vi "Metronome.vi"(8 "error in (no error)":errorcluster, 9 "MetronomeData":T2={"Interval"=250, "Message"="Tick"}, 10 "Queue in (write)":T1, 11 "Queue in (read)":T1) -> (0 "error out":errorcluster, 2 "Queue out (write)":T1, 3 "Queue out (read)":T1)   [LabVIEW 2020]
doc: "This VI enqueues a message with specified time interval in Queue in (write) queue. \nIt requires two refnums to queues made with CreateMessageQueue.vi. \nIt reads messages from Queue in (read). Valid messages: Start, Set, Pause, Stop. \nStart - begin or resume operations; Set - new interval (integer) provided as data with a message; Pause - halt operations and wait; Stop - stop VI.\nCluster MetronomeData provides an initial interval and text of the message to be send out in Queue in (write)."
uses:
  MetronomeData.ctl
  MessageQueue/QueueRef.ctl
  <vilib>/Utility/error.llb/Error Cluster From Error Code.vi
  <vilib>/ErrorRing/Error Ring.xnode
  MessageQueue/MessageQueue.lvlib
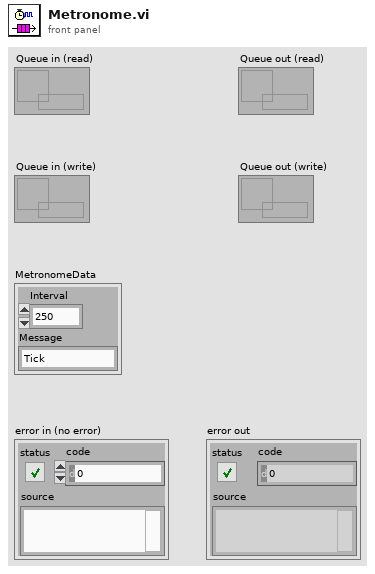
[diagram p1: front panel]
types:
  T1 = typedef "MessageQueue.lvlib/QueueRef.ctl" = refnum<queue>
  T2 = typedef "MetronomeData.ctl" = cluster{"Interval":i32, "Message":string}
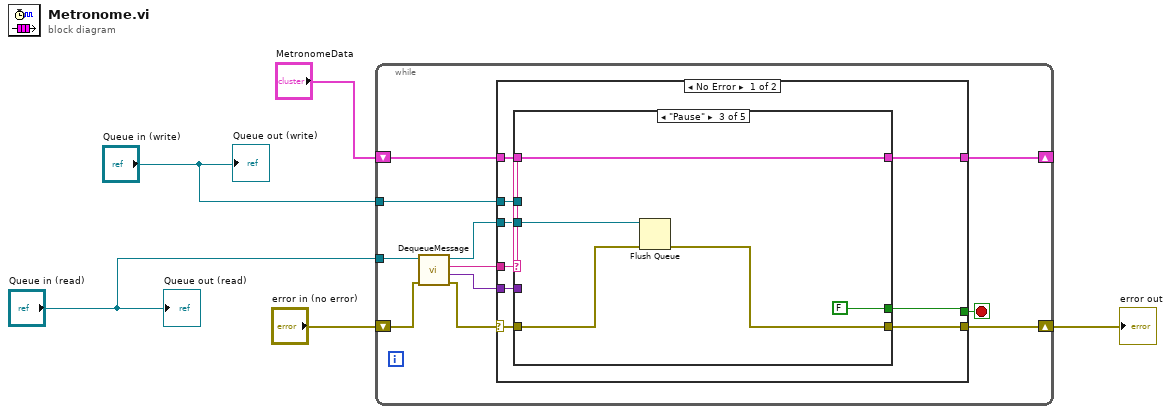
[diagram p0: block diagram]
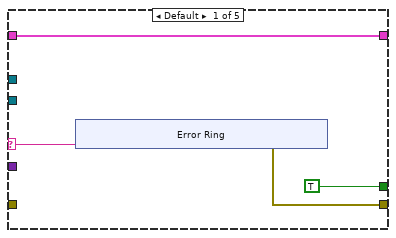
[diagram p2: hidden frame]
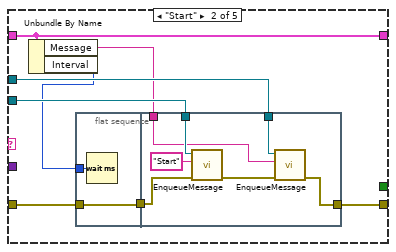
[diagram p3: hidden frame]
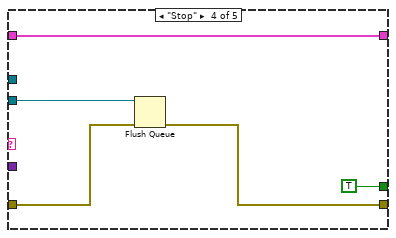
[diagram p4: hidden frame]
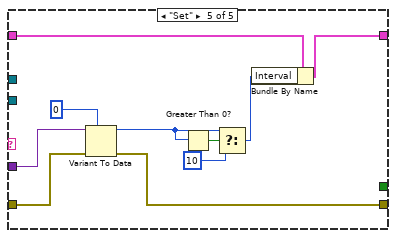
[diagram p5: hidden frame]
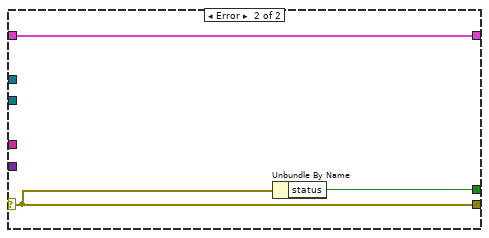
[diagram p6: hidden frame]
diagram:
  n1 = while {
    tunnel: "Queue in (read)" -> [w11]
    tunnel: "Queue in (write)" -> [w12]
    shift-right: [w15] -> _
    shift-left: "MetronomeData" -> [w16]
    shift-right: [w14] -> w4
    shift-left: "error in (no error)" -> [w7]
    stop <- w13 stop-if-true
    n2 = call "DequeueMessage.vi"("error in (no error)"=w7, "queue in"=w11) -> ("error out"=w6:errorcluster, "Data (Variant)"=w10:variant, "Message"=w9:string, "queue out (copy)"=w8:T1)  [unwired: 6 in]
    n3 = case shown="No Error" w6 {
      selector: w6 -> [w24 w75]
      tunnel: w16 -> [w23 w76]
      tunnel: [w22 w76] -> w15
      tunnel: [w25 w75] -> w14
      tunnel: [w20 w74] -> w13
      tunnel: w12 -> [w21 _]
      tunnel: w10 -> [w19 _]
      tunnel: w9 -> [w18 _]
      tunnel: w8 -> [w17 _]
      frame No Error {
        n4 = case shown="\"Pause\"" w18 {
          selector: w18 -> [w26 _ _ _ _]
          tunnel: [w27 w43 w56 w59 w67] -> w25
          tunnel: w24 -> [_ w37 w57 w62 w71]
          tunnel: w23 -> [w29 w41 w55 w61 w66]
          tunnel: [w29 w41 w55 w61 w65] -> w22
          tunnel: w17 -> [_ w44 w58 w63 _]
          tunnel: w21 -> [_ w42 _ _ _]
          tunnel: w19 -> [_ _ _ _ w73]
          tunnel: [TRUE _ FALSE TRUE _] -> w20
          frame Default {
            n5 = xnode "Error Ring"("parameter 0"=w26) -> ("error out"=w27:errorcluster)
          }
          frame "Start" {
            n6 = Unbundle By Name(w41) -> ("Message"=w39:string, "Interval"=w40:i32)
            n7 = flat-sequence {
              tunnel: w40 -> [w46]
              tunnel: [w45] -> w38
              tunnel: w37 -> [w45]
              tunnel: w44 -> [w52]
              tunnel: [w49] -> w43
              tunnel: w42 -> [w51]
              tunnel: w39 -> [w48]
              tunnel: w38 -> [w47]
              frame #0 {
                n8 = Wait (ms)(milliseconds to wait=w46) -> ()  [unwired: 1 out]
              }
              frame #1 {
                n9 = call "EnqueueMessage.vi"("error in (no error)"=w47, "Message"="Start", "queue in"=w52) -> ("error out"=w50:errorcluster)  [unwired: 7 in, 1 out]
                n10 = call "EnqueueMessage.vi"("error in (no error)"=w50, "Message"=w48, "queue in"=w51) -> ("error out"=w49:errorcluster)  [unwired: 7 in, 1 out]
              }
            }
          }
          frame "Pause" {
            n11 = Flush Queue(queue=w58, error in (no error)=w57) -> (error out=w56:errorcluster)  [unwired: 2 out]
          }
          frame "Stop" {
            n12 = Flush Queue(queue=w63, error in (no error)=w62) -> (error out=w59:errorcluster)  [unwired: 2 out]
          }
          frame "Set" {
            n13 = Variant To Data(error in=w71, type=0, Variant=w73) -> (data=w69:i32, error out=w67:errorcluster)
            n14 = Greater Than 0?(x=w69) -> (x > 0?=w70:bool)
            n15 = Select(t=w69, s=w70, f=10) -> (s? t:f=w64:i32)
            n16 = Bundle By Name(cluster=w66, "Interval"=w64) -> (w65:T2)
          }
        }
      }
      frame Error {
        n17 = Unbundle By Name(w75) -> ("status"=w74:bool)
      }
    }
  }
  "error out" <- w4
  "Queue out (write)" <- "Queue in (write)"
  "Queue out (read)" <- "Queue in (read)"
